vi "Set prefix.vi"(8 "error in (no error)":errorcluster, 10 "prefix":string="OBJ", 11 "Object DAO in":refnum<class "Object DAO.lvclass">) -> (0 "error out":errorcluster, 3 "Object DAO out":refnum<class "Object DAO.lvclass">)   [LabVIEW 2020, in "Object DAO.lvclass"]
uses:
  Object DAO.lvclass
  Object DAO.lvclass/Object DAO.ctl
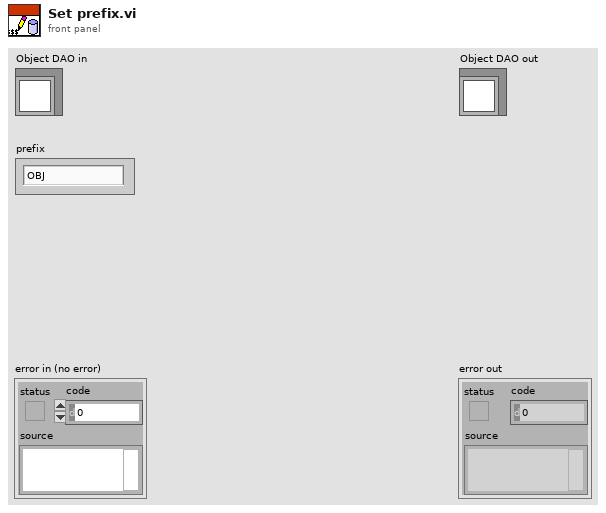
[diagram p1: front panel]
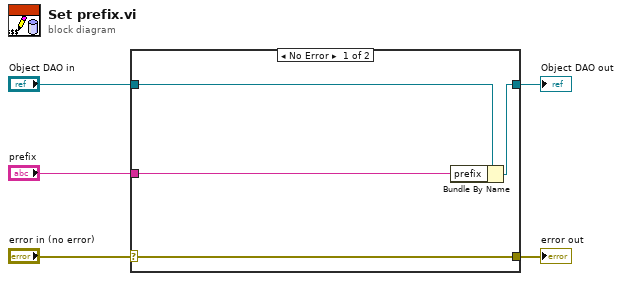
[diagram p0: block diagram]
diagram:
  n1 = case shown="No Error" "error in (no error)" {
    selector: "error in (no error)" -> [w9 w10]
    tunnel: [w9 w10] -> w4
    tunnel: [w7 w11] -> w2
    tunnel: "Object DAO in" -> [w8 w11]
    tunnel: "prefix" -> [w6 _]
    frame No Error {
      n2 = Bundle By Name(cluster=w8, "prefix"=w6) -> (w7:refnum<class "Object DAO.lvclass">)
    }
    frame Error {
    }
  }
  "error out" <- w4
  "Object DAO out" <- w2
